vi "DecodeBMPString.vi"(4 "error in":errorcluster, 6 "Compressed Image":string, 7 "Image In":T1) -> (0 "error out":errorcluster, 3 "Image Out":T1)   [LabVIEW 2017]
uses:
  <vilib>/vision/Image Controls.llb/IMAQ Image.ctl
panel:
  # "NEEDED: get image size from stream instead of 320x240 constant.\nHandle HTTP errors\nReverse rows, not entire array, currently HMirror.\nUse BuildCGI subVI"
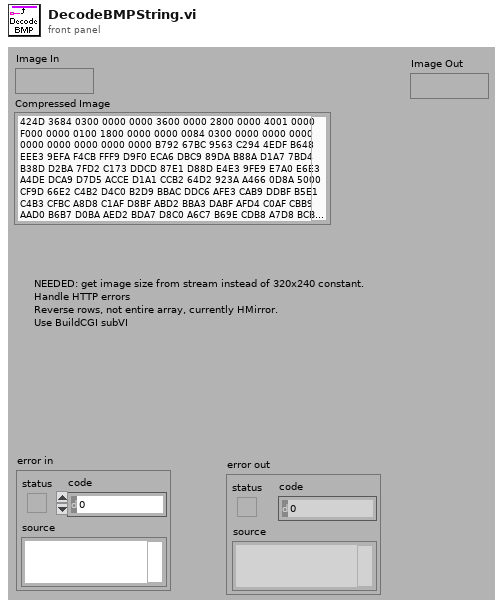
[diagram p1: front panel]
types:
  T1 = typedef "IMAQ Image.ctl" = refnum<image>
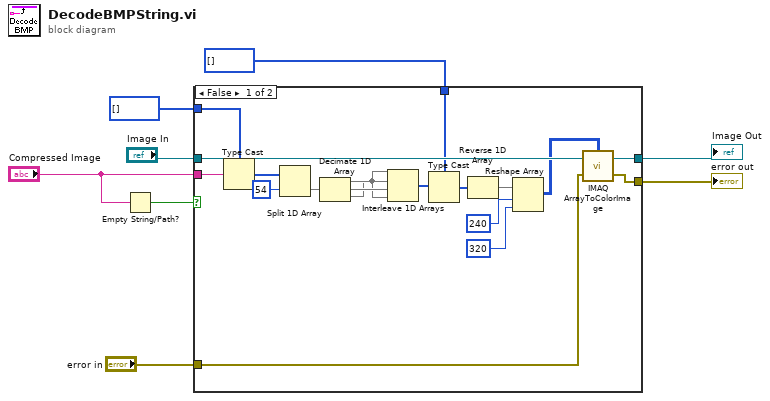
[diagram p0: block diagram]
diagram:
  n1 = Empty String/Path?(string/path="Compressed Image") -> (empty?=w3:bool)
  n2 = case shown="False" w3 {
    tunnel: "Compressed Image" -> [w27 _]
    tunnel: "Image In" -> [w23 w29]
    tunnel: "error in" -> [w21 w28]
    tunnel: [w20 w28] -> w6
    tunnel: [w22 w29] -> w5
    tunnel: u8[] [] -> [w26 _]
    tunnel: u32[] [] -> [w16 _]
    frame False {
      n3 = Type Cast(type=w26, x=w27) -> (*(type *) &x=w25:u8[])
      n4 = Split 1D Array(array=w25, index=54) -> (second subarray=w19:u8[])  [unwired: 1 out]
      n5 = Decimate 1D Array(w19) -> (w11:u8[], w18:u8[], w10:u8[])
      n6 = Interleave 1D Arrays(w11, w10, w18, w11) -> (w17:u8[])
      n7 = Type Cast(type=w16, x=w17) -> (*(type *) &x=w15:u32[])
      n8 = Reverse 1D Array(array=w15) -> (reversed array=w9:u32[])
      n9 = Reshape Array(w9, 240 ("index"), 320 ("index")) -> (w12:u32[][])
      n10 = call "IMAQ ArrayToColorImage"("Image Pixels (U32)"=w12, "Image"=w23, "error in (no error)"=w21) -> ("Image Out"=w22:T1, "error out"=w20:errorcluster)  [unwired: 2 in]
    }
    frame True {
    }
  }
  "error out" <- w6
  "Image Out" <- w5
